vi "Get Rack Info.vi"(11 "error in (no error)":errorcluster) -> (4 "Rack Info":string, 15 "error out":errorcluster)   [LabVIEW 2018]
uses:
  Station/GLOBALS.vi
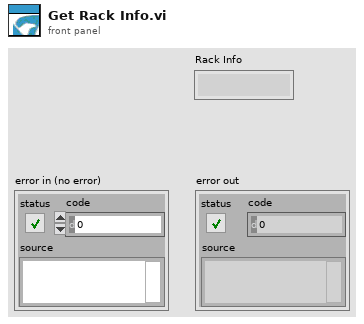
[diagram p1: front panel]
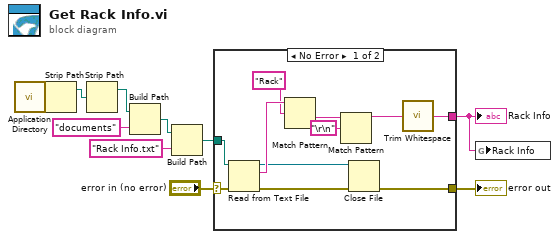
[diagram p0: block diagram]
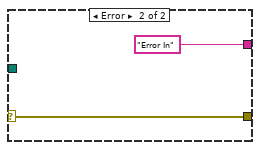
[diagram p2: hidden frame]
diagram:
  n1 = call <vilib>:"Application Directory.vi"() -> ("Application Directory"=w7:path)
  n2 = Strip Path(path=w7) -> (stripped path=w4:path)  [unwired: 1 out]
  n3 = Strip Path(path=w4) -> (stripped path=w3:path)  [unwired: 1 out]
  n4 = Build Path(base path=w3, name or relative path="documents") -> (appended path=w1:path)
  n5 = Build Path(base path=w1, name or relative path="Rack Info.txt") -> (appended path=w5:path)
  n6 = case shown="No Error" "error in (no error)" {
    selector: "error in (no error)" -> [w21 w23]
    tunnel: [w12 w23] -> w9
    tunnel: w5 -> [w20 _]
    tunnel: [w11 "Error In"] -> w8
    frame No Error {
      n7 = Read from Text File(file (use dialog)=w20, error in=w21) -> (refnum out=w13:refnum<file>, text=w19:string, error out=w14:errorcluster)  [unwired: 2 in, 1 out]
      n8 = Match Pattern(string=w19, regular expression="Rack") -> (after substring=w17:string)  [unwired: 1 in, 3 out]
      n9 = Match Pattern(string=w17, regular expression="\r\n") -> (before substring=w15:string)  [unwired: 1 in, 3 out]
      n10 = Close File(refnum=w13, error in=w14) -> (error out=w12:errorcluster)  [unwired: 1 out]
      n11 = call <vilib>:"Trim Whitespace.vi"("string"=w15) -> ("trimmed string"=w11:string)  [unwired: 1 in]
    }
    frame Error {
    }
  }
  "error out" <- w9
  "Rack Info" <- w8
  n12 = global write "GLOBALS.vi" "Rack Info"(w8) -> ()
